vi "Apply Application Style.vi"(8 "error in (no error)":errorcluster, 10 "VI Refnum":refnum<vi>, 11 "TestApplicationStyle in":refnum<class "TestApplicationStyle.lvclass">) -> (0 "error out":errorcluster)   [LabVIEW 2017, in "Integration Test Launcher.lvlib" / "TestApplicationStyle.lvclass"]
doc: "<License>\nCopyright © 2020 Tymphany, LLC | All rights reserved\nwww.Tymphany.com\nHuijun <Huijun.Guo@Tymphany.com>\n</License>"
uses:
  <vilib>/gpm_packages/@cs/example/Integration Test/TestApplicationStyle/TestApplicationStyle.lvclass
  <vilib>/gpm_packages/@cs/example/Integration Test/TestApplicationStyle/TestApplicationStyle.lvclass/TestApplicationStyle.ctl
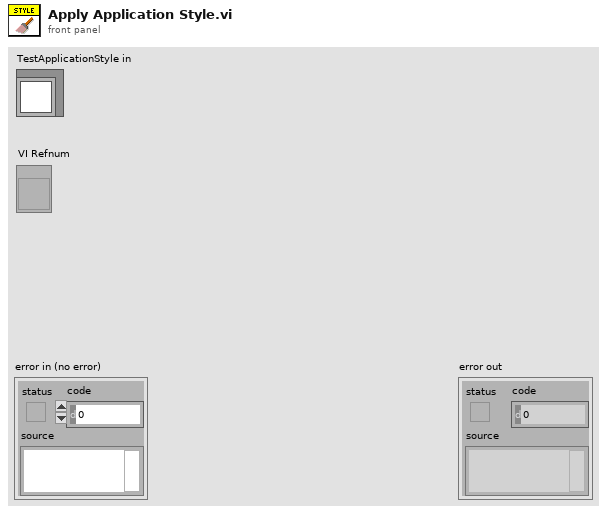
[diagram p1: front panel]
types:
  T1 = cluster{"Splitter Color":u32, "Splitter Color":u32}
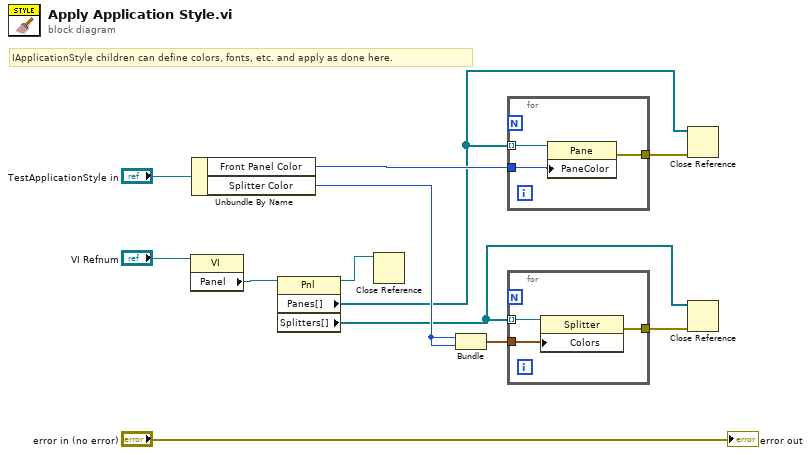
[diagram p0: block diagram]
diagram:
  # "IApplicationStyle children can define colors, fonts, etc. and apply as done here."
  n1 = property class="VI"(reference="VI Refnum") -> ("Panel"=w11:refnum<vi>)  [unwired: 1 in, 2 out]
  n2 = Unbundle By Name("TestApplicationStyle in") -> ("Front Panel Color"=w8:u32, "Splitter Color"=w6:u32)
  n3 = property class="Pnl"(reference=w11) -> (reference out=w1:refnum<vi>, "Panes[]"=w3:refnum<vi>[], "Splitters[]"=w2:refnum<vi>[])  [unwired: 1 in, 1 out]
  n4 = Close Reference(reference=w1) -> ()  [unwired: 1 in, 1 out]
  n5 = Bundle("Splitter Color"=w6, "Splitter Color"=w6) -> (w7:T1)  [unwired: 1 in]
  n6 = for {
    tunnel: w3 -> [w15] mode=indexing
    tunnel: w8 -> [w14]
    tunnel: [w13] -> w4
    n7 = property class="Pane"(reference=w15, "PaneColor"=w14) -> (error out=w13:errorcluster)  [unwired: 1 in, 1 out]
  }
  n8 = for {
    tunnel: w2 -> [w18] mode=indexing
    tunnel: w7 -> [w17]
    tunnel: [w16] -> w5
    n9 = property class="Splitter"(reference=w18, "Colors"=w17) -> (error out=w16:errorcluster)  [unwired: 1 in, 1 out]
  }
  n10 = Close Reference(reference=w3, error in (no error)=w4) -> ()  [unwired: 1 out]
  n11 = Close Reference(reference=w2, error in (no error)=w5) -> ()  [unwired: 1 out]
  "error out" <- "error in (no error)"
